vi "Write Steering Command Message.vi"(8 "error in (no error)":errorcluster, 10 "Steering Command Control":T1, 11 "Steering Command in":refnum<class "Steering Command.lvclass">) -> (0 "error out":errorcluster, 3 "Steering Command out":refnum<class "Steering Command.lvclass">)   [LabVIEW 2015, in "RDS Child Messages.lvlib" / "Steering Command.lvclass"]
uses:
  Steering Command.lvclass
  Steering Command Cntrl.ctl
  Steering Command.lvclass/Steering Command.ctl
  RDS Child Messages.lvlib
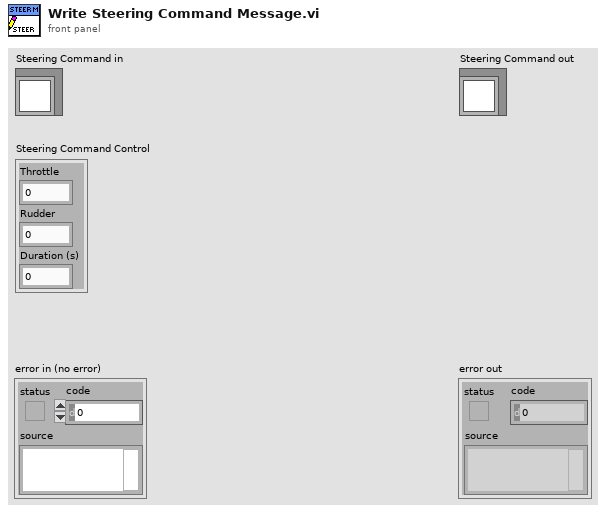
[diagram p1: front panel]
types:
  T1 = typedef "RDS Child Messages.lvlib/Steering Command Cntrl.ctl" = cluster{"Throttle":i16, "Rudder":i8, "Duration (s)":u16}
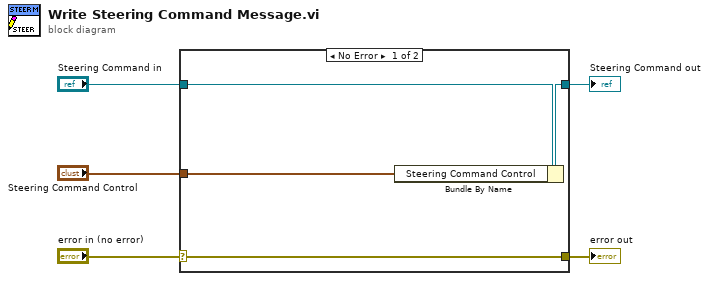
[diagram p0: block diagram]
diagram:
  n1 = case shown="No Error" "error in (no error)" {
    selector: "error in (no error)" -> [w9 w10]
    tunnel: [w9 w10] -> w4
    tunnel: [w7 w11] -> w2
    tunnel: "Steering Command in" -> [w8 w11]
    tunnel: "Steering Command Control" -> [w6 _]
    frame No Error {
      n2 = Bundle By Name(cluster=w8, "Steering Command Control"=w6) -> (w7:refnum<class "Steering Command.lvclass">)
    }
    frame Error {
    }
  }
  "error out" <- w4
  "Steering Command out" <- w2
